vi "cluster.vi"(11 "Input":cluster{"gain":dbl, "Array":dbl[]}={"gain"=1.0, "Array"=[2.0]}) -> (3 "Output":cluster{"Array":dbl[], "sum":dbl}={"Array"=[3.0], "sum"=4.0})   [LabVIEW 2020]
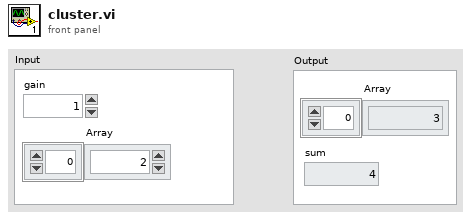
[diagram p1: front panel]
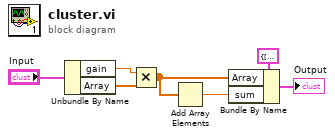
[diagram p0: block diagram]
diagram:
  n1 = Unbundle By Name("Input") -> ("gain"=w6:dbl, "Array"=w5:dbl[])
  n2 = Multiply(x=w6, y=w5) -> (x*y=w4:dbl[])
  n3 = Add Array Elements(numeric array=w4) -> (sum=w1:dbl)
  n4 = Bundle By Name(cluster=cluster{"Array":dbl[], "sum":dbl} {"Array"=[], "sum"=0.0} ("Output"), "Array"=w4, "sum"=w1) -> (→"Output":cluster{"Array":dbl[], "sum":dbl})
